vi "AvgArrayData.vi"() -> ()   [LabVIEW 2022 SP3]
uses:
  <vilib>/Analysis/NI_AALBase.lvlib
  <vilib>/Analysis/baseanly.llb/Mean (DBL).vi
panel:
  in  "save?":bool
  out "Raw data":dbl[][](graph)
  in  "Display mode":u16(ring)=1 items=["Linear Abs Grey", "Log Grey Scale", "Linear Color Scale"]
  in  "# in set":i32=25
  out "Current File":string
  in  "Use Selected Files":bool
  in  "Listbox":i32[](listbox)
  in  "file ext":string="*1to1*"
  in  "Folder to save in":path=path "D:/Temp/AVG"
  in  "Folder with files":path=path "D:/Temp"
  in  "# to planes":i32
  in  "Ring":u16(ring) items=["Annular Array", "2-D Scans", "List box"]
  out "Array":string[](array[string])
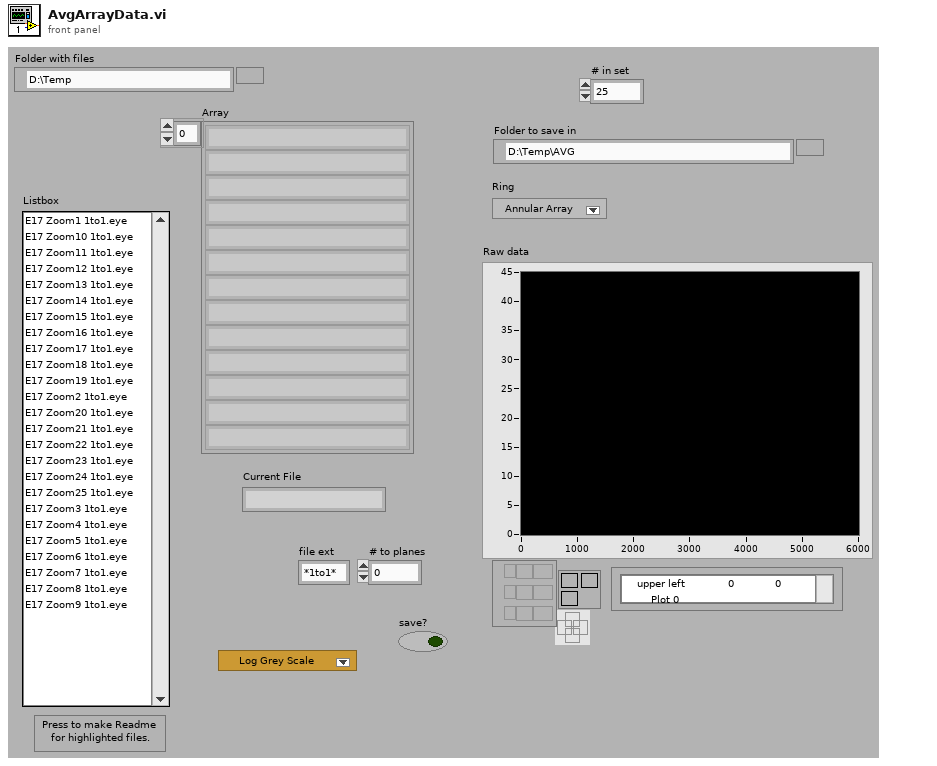
[diagram p1: front panel]
types:
  T1 = typedef "Header.ctl" = cluster{"header info":cluster{"Header":string, "Head length":i16}, "A/D info":cluster{"# rf points per line":u16, "# lines per scan":u16, "sample rate MHz":u16, "# A/D bits":i16, "# bytes per A/D":u16, "TGC Flag":u16, "A/D Type":string}, "Tranducer Info":cluster{"bandwidth":sgl, "center freq":sgl, "start freq":sgl, "ID":i32}, "Scan Info":cluster{"delay":sgl, "pivot distance":sgl, "sector scan angle":sgl, "operator":string, "Scan Mode":string, "location":string}, "Time/Date Info":cluster{"date":string, "time":string}, "RF Info":cluster{"RF file name":string, "RF file att":string, "RF cal file name":string, "RF cal file att":string}, "Patient Info":cluster{"ID":string, "extended ID":string, "age":u16, "sex":string, "previously\nscanned":string, "PSA":sgl, "LOS":u8, "Ethnicty 2":u8, "Race":u8}, "Tissue Type":cluster{"organ":i16, "disease type":i16, "disease location":i16, "IQ_pts":u16, "RcvBuffer":u8, "RcvFrame":u16, "IQBuff":u8, "IQFrame":u16, "IQPage":u8}, "Votage scaling":cluster{"Digitizer (dB)":sgl, "Gain (dB)":sgl, "Atten (dB)":sgl}, "Comment":string, "Misc Info":cluster{"avg num":u16, "c speed":i16, "Div By or SF zones":i16, "XMIT CHS":u8, "RCV CHS":u8, "Xmit angle":sgl}, "Therapy Parameters":cluster{"Theraputic Freq (MHz)":sgl, "Time on (s)":sgl, "Therapy amplitude (mV)":sgl, "Lines Before":u16, "Lines After":u16}, "Scan Settings":cluster{"Energy (uJ or V)":u8, "Damp (Ohm) or Fc":u8, "HP Filt (KHz)":u8, "LP Filt (MHz)":u8, "Gain (db)":u8, "prf (kHz)":sgl, "Distance between\nscan lines (um)":u16, "Distance between\nscan planes (um)":u16, "Scan line gap (um)":sgl, "Scan plane gap (um)":sgl}, "Compression Parameters":cluster{"F1 (MHz)":sgl, "F2 (MHz)":sgl, "% taper":sgl, "duration":sgl}, "Patient Info Xtra":cluster{"First Name":string, "Last Name":string, "Notes":string}, "ROI Box":u16[]}
  T2 = cluster{"# rf points per line":u16, "# lines per scan":u16, "sample rate MHz":u16, "# A/D bits":u16, "# bytes per A/D":u16, "TGC Flag":u16, "A/D Type":string}
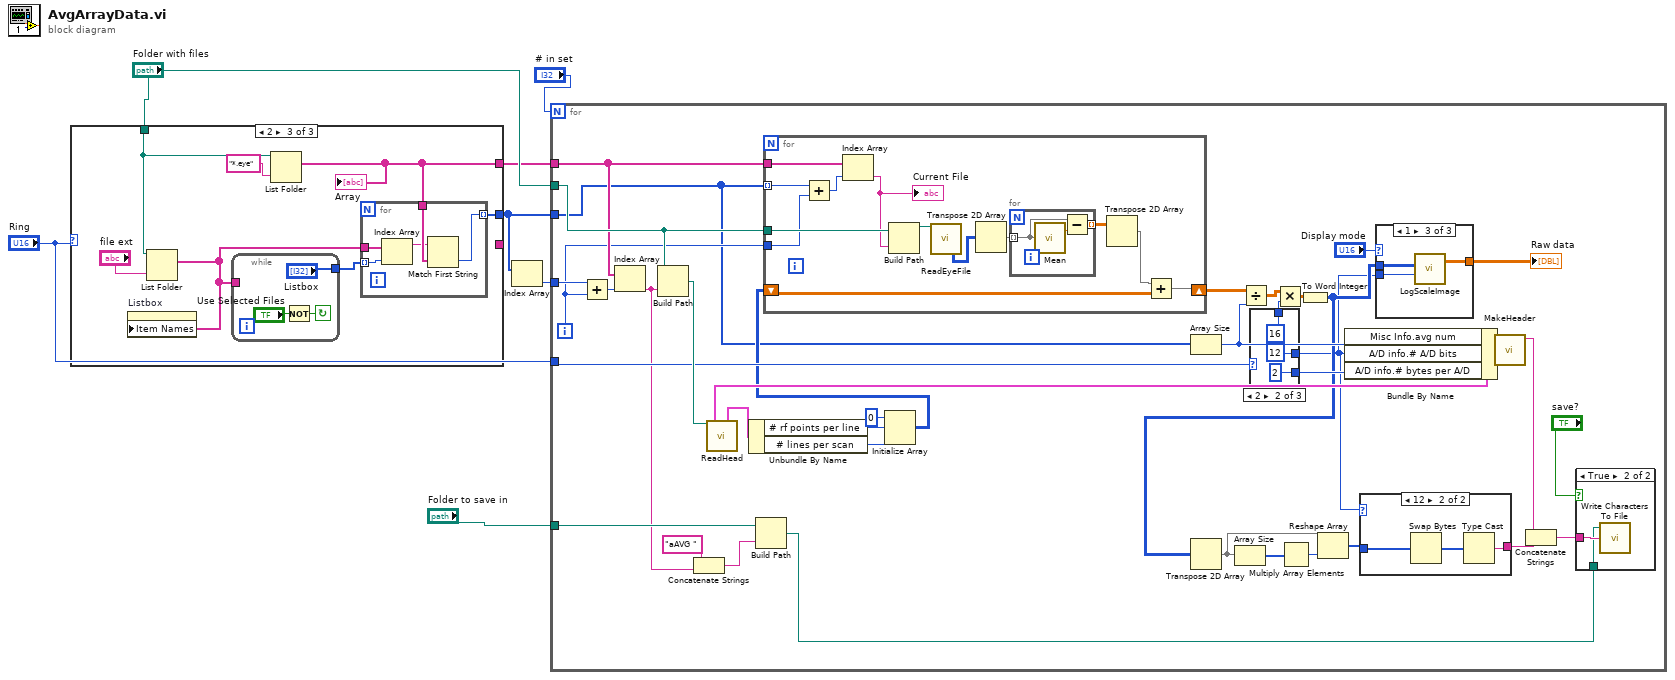
[diagram p0: block diagram]
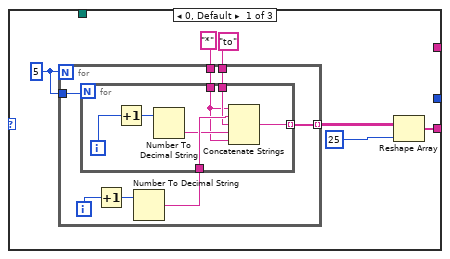
[diagram p2: hidden frame]
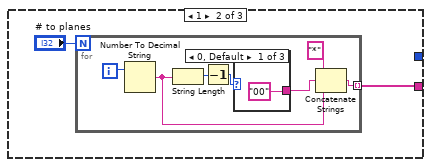
[diagram p3: hidden frame]
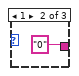
[diagram p4: hidden frame]
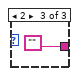
[diagram p5: hidden frame]
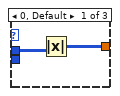
[diagram p6: hidden frame]
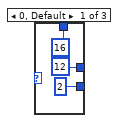
[diagram p8: hidden frame]
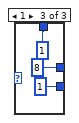
[diagram p9: hidden frame]
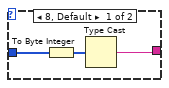
[diagram p10: hidden frame]
diagram:
  n1 = case shown="2" "Ring" {
    tunnel: [w8 w28 _] -> _
    tunnel: "Folder with files" -> [_ _ w45]
    tunnel: [_ _ w40] -> w4
    tunnel: [_ _ w41] -> w3
    frame 0, Default {
      w11 = 5
      n2 = for {
        N: w11 -> [_]
        tunnel: "*" -> [w18]
        tunnel: "to" -> [w16]
        tunnel: w11 -> [w15]
        tunnel: [w14] -> w10 mode=indexing
        i -> [w20]
        n3 = Increment(x=w20) -> (x+1=w19:i32)
        n4 = Number To Decimal String(number=w19) -> (decimal integer string=w17:string)  [unwired: 1 out]
        n5 = for {
          N: w15 -> [_]
          tunnel: w18 -> [w22]
          tunnel: w17 -> [w25]
          tunnel: w16 -> [w24]
          tunnel: [w21] -> w14 mode=indexing
          i -> [w26]
          n6 = Increment(x=w26) -> (x+1=w27:i32)
          n7 = Number To Decimal String(number=w27) -> (decimal integer string=w23:string)  [unwired: 1 out]
          n8 = Concatenate Strings(w22, w25, w24, w23, w22) -> (w21:string)
        }
      }
      n9 = Reshape Array(w10, 25) -> (w8:string[])
    }
    frame 1 {
      n10 = for {
        N: "# to planes" -> [_]
        tunnel: [w33] -> w28 mode=indexing
        i -> [w36]
        n11 = Number To Decimal String(number=w36) -> (decimal integer string=w31:string)  [unwired: 1 out]
        n12 = String Length(string=w31) -> (length=w34:i32)
        n13 = Decrement(x=w34) -> (x-1=w35:i32)
        n14 = case shown="0, Default" w35 {
          tunnel: ["00" "0" ""] -> w30
          frame 0, Default {
          }
          frame 1 {
          }
          frame 2 {
          }
        }
        n15 = Concatenate Strings("*", w30, w31) -> (w33:string)
      }
    }
    frame 2 {
      n16 = List Folder(path=w45, pattern="file ext") -> (filenames=w42:string[])  [unwired: 1 in, 4 out]
      n17 = property on="Listbox" class="LstBox (strict)"("Item Names"=w42) -> ()  [unwired: 2 in, 2 out]
      n18 = while {
        tunnel: ["Listbox"] -> w43
        tunnel: w42 -> [_]
        stop <- w54 continue-if-true
        n19 = Not(x="Use Selected Files") -> (.not. x?=w54:bool)
      }
      n20 = List Folder(path=w45, pattern="*.eye") -> (filenames=w40:string[])  [unwired: 1 in, 4 out]
      "Array" <- w40
      n21 = for {
        tunnel: w43 -> [w51] mode=indexing
        tunnel: w42 -> [w49]
        tunnel: w40 -> [w50]
        tunnel: [w47] -> w41 mode=indexing
        n22 = Index Array(array=w49, index=w51) -> (element=w48:string)
        n23 = Match First String(2:w50, 3:w48) -> (0:w47:i32)  [unwired: 1 out]
      }
    }
  }
  n24 = Index Array(array=w3) -> (element=w2:i32)  [unwired: 1 in]
  n25 = for {
    N: "# in set" -> [_]
    tunnel: "Folder with files" -> [w69]
    tunnel: "Folder to save in" -> [w77]
    tunnel: "Ring" -> [w70]
    tunnel: w4 -> [w67]
    tunnel: w3 -> [w55]
    tunnel: w2 -> [w66]
    i -> [w63]
    n26 = Add(x=w66, y=w63) -> (x+y=w68:i32)
    n27 = Index Array(array=w67, index=w68) -> (element=w58:string)
    n28 = Build Path(base path=w69, name or relative path=w58) -> (appended path=w92:path)
    n29 = Concatenate Strings("aAVG ", w58) -> (w57:string)
    n30 = call "ReadHead.vi"("new file path"=w92) -> ("Header In"=w85:T1, "A/D info"=w65:T2)  [unwired: 17 out]
    n31 = Unbundle By Name(w65) -> ("# rf points per line"=w87:u16, "# lines per scan"=w86:u16)
    n32 = Build Path(base path=w77, name or relative path=w57) -> (appended path=w76:path)
    n33 = Initialize Array(0, w87, w86) -> (w64:i32[][])
    n34 = for {
      tunnel: w69 -> [w128]
      shift-right: [w125] -> w91
      shift-left: w64 -> [w126]
      tunnel: w67 -> [w119]
      tunnel: w55 -> [w118] mode=indexing
      tunnel: w63 -> [w117]
      n35 = Add(x=w118, y=w117) -> (x+y=w120:i32)
      n36 = Index Array(array=w119, index=w120) -> (element=w116:string)
      "Current File" <- w116
      n37 = Build Path(base path=w128, name or relative path=w116) -> (appended path=w127:path)
      n38 = call "ReadEyeFile.vi"("new file path"=w127) -> ("2-D data array"=w122:i16[][])  [unwired: 1 in, 17 out]
      n39 = Transpose 2D Array(2D array=w122) -> (transposed array=w124:i16[][])
      n40 = for {
        tunnel: [w130] -> w123 mode=indexing
        tunnel: w124 -> [w129] mode=indexing
        n41 = call-poly <vilib>:"Mean.vi"("X"=w129) -> ("mean"=w131:dbl)  [unwired: 1 out]
        n42 = Subtract(x=w129, y=w131) -> (x-y=w130:dbl[])
      }
      n43 = Transpose 2D Array(2D array=w123) -> (transposed array=w121:dbl[][])
      n44 = Add(x=w121, y=w126) -> (x+y=w125:dbl[][])
    }
    n45 = Array Size(array=w55) -> (size(s)=w90:i32)
    n46 = Divide(x=w91, y=w90) -> (x/y=w74:dbl[][])
    n47 = case shown="2" w70 {
      tunnel: [2 2 1] -> w72
      tunnel: [16 16 1] -> w71
      tunnel: [12 12 8] -> w61
      frame 0, Default {
      }
      frame 2 {
      }
      frame 1 {
      }
    }
    n48 = Multiply(x=w74, y=w71) -> (x*y=w73:dbl[][])
    n49 = To Word Integer(number=w73) -> (16bit integer=w62:i16[][])
    n50 = Transpose 2D Array(2D array=w62) -> (transposed array=w75:i16[][])
    n51 = Array Size(array=w75) -> (size(s)=w81:i32[])
    n52 = Multiply Array Elements(1:w81) -> (0:w80:i32)
    n53 = Reshape Array(w75, w80) -> (w79:i16[])
    n54 = Bundle By Name(cluster=w85, "Misc Info.avg num"=w90, "A/D info.# A/D bits"=w61, "A/D info.# bytes per A/D"=w72) -> (w89:T1)
    n55 = case shown="12" w61 {
      tunnel: w79 -> [w109 w112]
      tunnel: [w110 w113] -> w83
      frame 8, Default {
        n56 = To Byte Integer(number=w109) -> (8bit integer=w108:i8[])
        n57 = Type Cast(x=w108) -> (*(type *) &x=w110:string)  [unwired: 1 out]
      }
      frame 12 {
        n58 = Swap Bytes(anything=w112) -> (byte swapped=w111:i16[])
        n59 = Type Cast(x=w111) -> (*(type *) &x=w113:string)  [unwired: 1 out]
      }
    }
    n60 = case shown="1" "Display mode" {
      tunnel: [w93 w95 w98] -> w59
      tunnel: w62 -> [w94 w95 w97]
      tunnel: w61 -> [_ _ w96]
      frame 0, Default {
        n61 = Absolute Value(x=w94) -> (abs(x)=w93:i16[][])
      }
      frame 2 {
      }
      frame 1 {
        n62 = call "LogScaleImage.vi"("A/D bits"=w96, "input array"=w97) -> ("log scale image"=w98:dbl[][])  [unwired: 1 out]
      }
    }
    "Raw data" <- w59
    n63 = call "MakeHeader.vi"("Header In"=w89) -> ("Header String"=w84:string)  [unwired: 6 out]
    n64 = Concatenate Strings(w84, w83) -> (w82:string)
    n65 = case shown="True" "save?" {
      tunnel: w82 -> [_ w115]
      tunnel: w76 -> [_ w114]
      frame False {
      }
      frame True {
        n66 = call <vilib>:"Write Characters To File.vi"("character string"=w115, "file path (dialog if empty)"=w114) -> ()  [unwired: 1 in, 3 out]
      }
    }
  }
